vi "Drive Controller.vi"(8 "error in":errorcluster) -> ()   [LabVIEW 2015]
doc: "This VI executes continuously carrying out the current operation and responding to updates or new operation requests. It will often contain the timing or control code that is difficult to place directly in TeleOp. This VI generally opens all sensors and motors and isolates the rest of the robot code from knowing implementation details of how the operations are carried out."
uses:
  Drive Operations.ctl
  Drive Setpoints.ctl
  <vilib>/Rock Robotics/WPI/SafetyOutput/WPI_SafetyOutputConfigMenu.ctl
  Support Code/Team900-VIs/navX/navX Library v2/navX Library v2.lvlib
  Support Code/Team900-VIs/Team900SwerveDrive/Team900SwerveDrive.lvlib
  <vilib>/Rock Robotics/WPI/RobotDrive/WPI_RobotDriveOpen4MotorWithCANTalonSRX.vi
  Support Code/Team900-VIs/navX/navX Library v2/IO/Open/Z900_navX_Open_SPI.vi
  <vilib>/Rock Robotics/SystemInterfaces/spilib/spi_bus.ctl
panel:
  out "Setpoints":T1(graph)
  out "Current\nCmd":string
  # "Tip: It may be helpful to observe inputs and sensor values.\nYou may also want to display tuning or debugging controls."
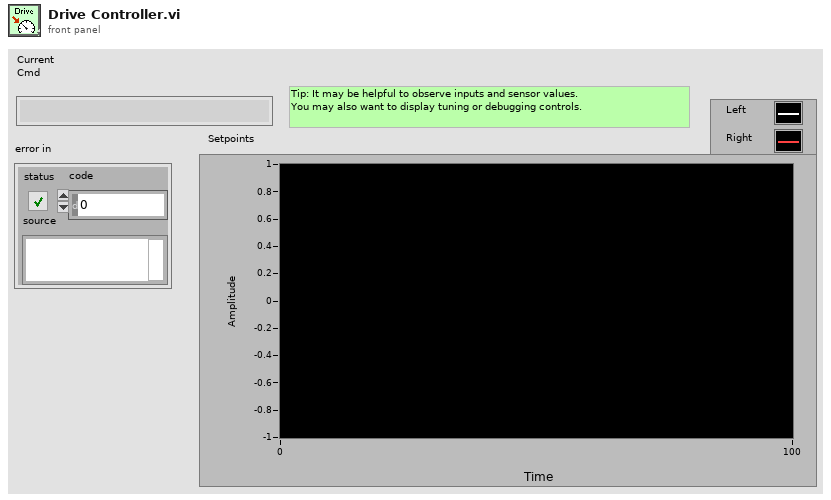
[diagram p1: front panel]
types:
  T1 = cluster{"Left Setpoint":dbl, "Right Setpoint":dbl}
  T2 = typedef "spi_bus.ctl" = enum16{"SPI On-Board, CS0", "SPI On-Board, CS1", "SPI On-Board, CS2", "SPI On-Board, CS3", "SPI MXP", "Invalid"}
  T3 = typedef "WPI_SafetyOutputConfigMenu.ctl" = enum16{"Enable", "Disable"}
  T4 = typedef "Drive Setpoints.ctl" = cluster{"Operation":T5, "Left Setpoint":dbl, "Right Setpoint":dbl, "Duration":dbl, "Straight Setpoint":dbl}
  T5 = typedef "Drive Operations.ctl" = enum16{"Reserve", "Read Current", "Immediate", "Drive for Time", "Drive for Distance", "Cross Defense"}
  T6 = typedef "WPI_RobotDriveDevRef.ctl" = cluster{"DevStatus":errorcluster, "Motors[]":T7[], "Square Inputs":bool, "Max Output":dbl}
  T7 = typedef "WPI_MotorControlDeviceRef.ctl" = cluster{"DeviceStatus":errorcluster, "Type":T8, "PWM":cluster{"PWM Channel":T9, "DeadBand":T10}, "CAN":cluster{"Device Number":u8, "Control Mode":T11, "Semaphore":T12, "Max Vout":dbl, "TalonSRX Control Mode":T13}, "Invert":bool}
  T8 = typedef "WPI_MotorControlType.ctl" = enum16{"PWM", "CAN", "CANTalonSRX"}
  T9 = typedef "FPGA_DIOPWMChannel.ctl" = enum8{"PWM 0", "PWM 1", "PWM 2", "PWM 3", "PWM 4", "PWM 5", "PWM 6", "PWM 7", "PWM 8", "PWM 9", "PWM MXP 0", "PWM MXP 1", "PWM MXP 2", "PWM MXP 3", "PWM MXP 4", "PWM MXP 5", "PWM MXP 6", "PWM MXP 7", "PWM MXP 8", "PWM MXP 9", "Invalid"}
  T10 = typedef "WPI_PWMDeadband.ctl" = cluster{"Name":string, "maxPositivePwm":i32, "minPositivePwm":i32, "centerPwm":i32, "maxNegativePwm":i32, "minNegativePwm":i32, "angularRange":u16}
  T11 = typedef "WPI_CANJaguar_ControlMode.ctl" = enum8{"Percent VBus", "Current", "Speed", "Position", "Voltage"}
  T12 = typedef "Semaphore RefNum" = refnum<k1>
  T13 = typedef "WPI_CANTalonSRX_APIControlMode.ctl" = enum8{"Percent VBus", "Speed", "Position", "Slave", "Unchanged / Invalid", "Voltage Compensation", "Current", "Motion Profile"}
  T14 = typedef "navX Library v2.lvlib/Z900_navX_DeviceTypeDef.ctl" = cluster{"Interface":cluster{"Protocol":T15, "Update Rate (4Hz-60Hz)":u8, "navX Open TypeDef":variant}, "Notify Packet":refnum<notifier>, "Loop VI Refnum":refnum<vi>, "Ready to Close Occurrence Refnum":refnum<k4>}
  T15 = typedef "navX Library v2.lvlib/Z900_navX_ProtocolTypeDef.ctl" = enum16{"SERIAL", "I2C", "SPI"}
  T16 = cluster{"Velocity X":dbl, "Velocity Y":dbl, "Velocity Z":dbl, "Displacement X":dbl, "Displacement Y":dbl, "Displacement Z":dbl}
  T17 = typedef "Command Status Info.ctl" = cluster{"Name":string, "Status":T18, "notifier out":T19}
  T18 = typedef "Completion Status.ctl" = enum16{"Successful", "Aborted", "Incomplete"}
  T19 = typedef "Completion Notifier.ctl" = refnum<notifier>
  T20 = cluster{"SubSystem Data":T4, cluster{"Start Time (ms)":u32, "Iterations":i32}, cluster{"Command Info":T17, "Description":string, "SubSystem Data":T4, "notifier out":refnum<notifier>, "Subsystem Name":string}}
  T21 = cluster{"Yaw":dbl, "Roll":dbl, "Pitch":dbl, "Heading":dbl, "Fused Heading":dbl}
  T22 = cluster{"Don't move motors while reserved":dbl, "Don't move motors while reserved":dbl}
  T23 = cluster{"SubSystem Data":T4, cluster{"Start Time (ms)":u32, "Iterations":i32}, "Default Command Arguments":cluster{"Command Info":T17, "Description":string, "SubSystem Data":T4, "notifier out":refnum<notifier>, "Subsystem Name":string}}
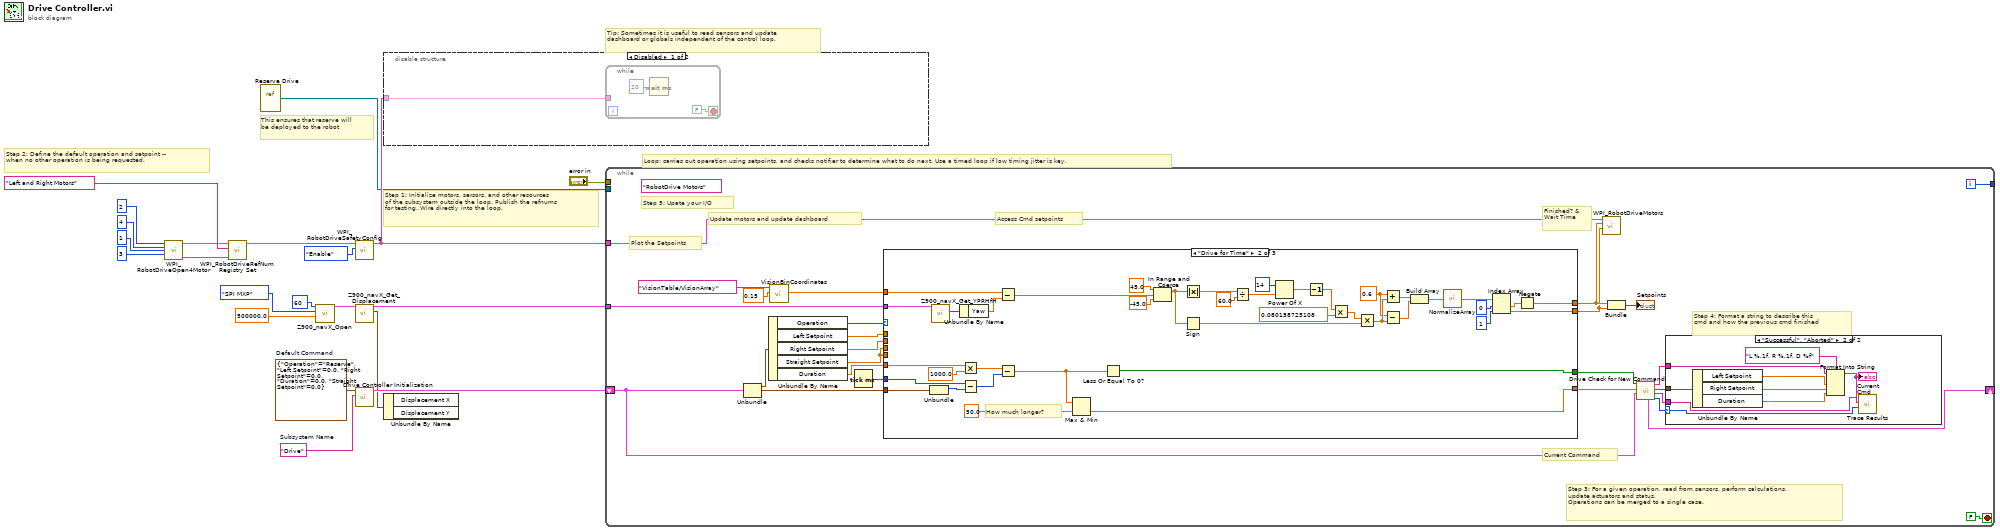
[diagram p0: block diagram]
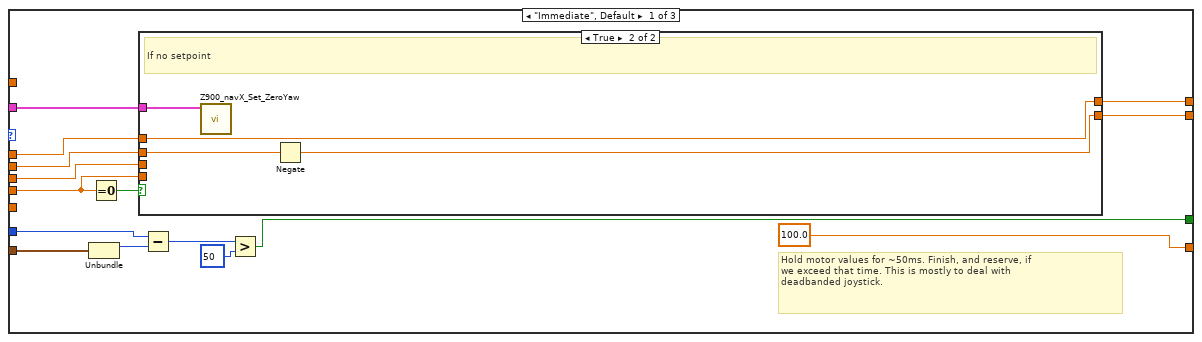
[diagram p4: hidden frame]
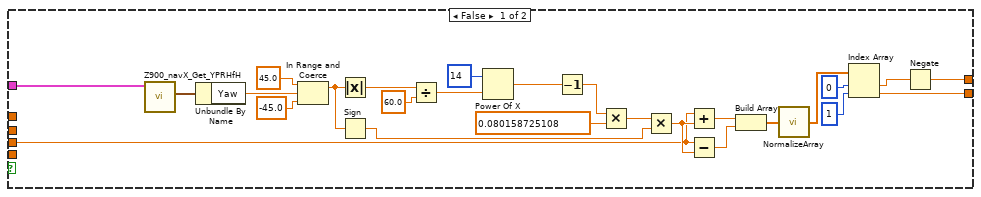
[diagram p5: hidden frame]
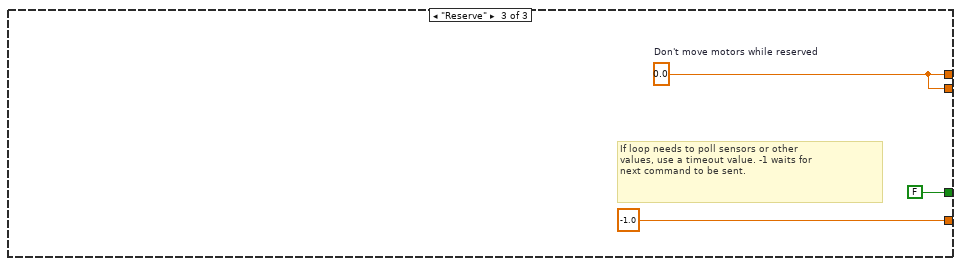
[diagram p6: hidden frame]
diagram:
  w20 = T4 {"Operation"=enum."Reserve", "Left Setpoint"=0.0, "Right Setpoint"=0.0, "Duration"=0.0, "Straight Setpoint"=0.0}  # Default Command
  w21 = "Drive"  # Subsystem Name
  # "This ensures that reserve will\nbe deployed to the robot"
  # "Tip: Sometimes it is useful to read sensors and update\ndashboard or globals independent of the control loop."
  # "Step 2: Define the default operation and setpoint --\nwhen no other operation is being requested."
  # "Step 1: Initialize motors, sersors, and other resources\nof the subsystem outside the loop. Publish the refnums\nfor testing. Wire directly into the loop."
  # "Loop: carries out operation using setpoints, and checks notifier to determine what to do next. Use a timed loop if low timing jitter is key."
  n1 = call-poly <vilib>:"WPI_RobotDriveOpen4Motor.vi"("Rear Left Motor"=u8 2, "Rear Right Motor"=u8 4, "Front Left Motor"=u8 1, "Front Right Motor"=u8 3) -> ("RobotDriveDevRef"=w12:T6, "error out"=w11:errorcluster)  [unwired: 10 in]
  n2 = call <vilib>:"WPI_RobotDriveRefNum Registry Set.vi"("error in (no error)"=w11, "refnum name"="Left and Right Motors", "RobotDriveDevRef"=w12) -> ("RobotDriveDevRef"=w18:T6)  [unwired: 1 in, 7 out]
  n3 = vi-ref "Reserve Drive.vi"() -> (w13:refnum<vi>)
  n4 = call-poly "Z900_navX_Open.vi"("Clock Rate (Hz)"=500000.0, "SPI Bus"=spi_bus."SPI MXP", "Update Rate (4Hz-60Hz)"=u8 60) -> ("navX Device"=w3:T14)  [unwired: 7 in, 1 out]
  n5 = call <vilib>:"WPI_RobotDriveSafetyConfig.vi"("mode"=WPI_SafetyOutputConfigMenu."Enable", "RobotDriveDevRef"=w18) -> ("RobotDriveDevRef"=w16:T6)  [unwired: 8 in, 1 out]
  n6 = call "Z900_navX_Get_Displacement.vi"("navX Device"=w3) -> ("Displacement"=w1:T16, "navX Device"=w2:T14)  [unwired: 7 in, 2 out]
  n7 = call "Drive Controller Initialization.vi"("Subsystem Name"=w21, "Default Command"=w20) -> ("output cluster"=w14:T20)  [unwired: 9 in]
  n8 = disable-structure shown="Disabled" {
    disable-tunnel: w16 -> [w22 _]
    frame Disabled {
      n9 = while {
        tunnel: w22 -> [_]
        stop <- FALSE stop-if-true
        n10 = Wait (ms)(milliseconds to wait=u32 20) -> ()  [unwired: 1 out]
      }
    }
    frame Enabled {
    }
  }
  n11 = Unbundle By Name(w1) -> ()  [unwired: 2 out]
  n12 = while {
    shift-right: [w38] -> _
    shift-left: w14 -> [w31]
    tunnel: [w49] -> _
    tunnel: w16 -> [w45]
    tunnel: "error in" -> [_]
    tunnel: w13 -> [_]
    tunnel: w2 -> [w28]
    i -> [w49]
    stop <- FALSE stop-if-true
    (unwired) "RobotDrive Motors" ("Name")
    # "Step 5: Upate your I/O"
    # "Step 4: Format a string to describe this\ncmd and how the previous cmd finished"
    # "Current Command"
    # "Update motors and update dashboard"
    # "Plot the Setpoints"
    # "Access Cmd setpoints"
    # "Finished? &\nWait Time"
    # "Step 3: For a given operation, read from sensors, perform calculations,\nupdate actuators and status.\nOperations can be merged to a single case."
    n13 = Unbundle(w31) -> ("SubSystem Data"=w44:T4, w32:cluster{"Start Time (ms)":u32, "Iterations":i32})  [unwired: 1 out]
    n14 = Unbundle By Name(w44) -> ("Operation"=w43:T5, "Left Setpoint"=w42:dbl, "Right Setpoint"=w41:dbl, "Straight Setpoint"=w29:dbl, "Duration"=w30:dbl)
    n15 = call "VisionBinCoordinates.vi"("Minimum Ratio"=0.15, "Vision Array Name"="VisionTable/VisionArray") -> ("bin angle"=w25:dbl)  [unwired: 2 in, 4 out]
    n16 = Tick Count (ms)() -> (millisecond timer value=w40:u32)
    n17 = case shown="\"Drive for Time\"" w43 {
      tunnel: [100.0 w134 -1.0] -> w37
      tunnel: [w69 w138 FALSE ("ignore previous (F)")] -> w36
      tunnel: w32 -> [w68 w140 _]
      tunnel: [w66 w110 w144] -> w47
      tunnel: [w64 w111 w144] -> w46
      tunnel: w42 -> [w65 _ _]
      tunnel: w41 -> [w63 _ _]
      tunnel: w29 -> [w62 _ _]
      tunnel: w40 -> [w70 w137 _]
      tunnel: w30 -> [_ w133 _]
      tunnel: w28 -> [w61 w108 _]
      tunnel: w29 -> [w60 _ _]
      tunnel: w25 -> [_ w105 _]
      frame "Immediate", Default {
        # "Hold motor values for ~50ms. Finish, and reserve, if\nwe exceed that time. This is mostly to deal with\ndeadbanded joystick."
        n18 = Unbundle(w68) -> ("Start Time (ms)"=w71:u32)  [unwired: 1 out]
        n19 = Equal To 0?(x=w62) -> (x = 0?=w67:bool)
        n20 = case shown="True" w67 {
          tunnel: [w80 w104] -> w66
          tunnel: w65 -> [_ w104]
          tunnel: [w81 w101] -> w64
          tunnel: w63 -> [_ w103]
          tunnel: w62 -> [_ _]
          tunnel: w61 -> [w100 w102]
          tunnel: w60 -> [w84 _]
          frame False {
            n21 = call "Z900_navX_Get_YPRHfH.vi"("navX Device"=w100) -> ("YRPHfH"=w83:T21)  [unwired: 7 in, 3 out]
            n22 = Unbundle By Name(w83) -> ("Yaw"=w76:dbl)
            n23 = In Range and Coerce(upper limit=45.0, x=w76, lower limit=-45.0) -> (coerced(x)=w75:dbl)  [unwired: 1 out]
            n24 = Absolute Value(x=w75) -> (abs(x)=w94:dbl)
            n25 = Sign(1:w75) -> (0:w92:dbl)
            n26 = Divide(x=w94, y=60.0) -> (x/y=w97:dbl)
            n27 = Power Of X(1:w97, 2:14) -> (0:w96:dbl)
            n28 = Decrement(x=w96) -> (x-1=w95:dbl)
            n29 = Multiply(x=w95, y=0.080158725108) -> (x*y=w93:dbl)
            n30 = Multiply(x=w93, y=w92) -> (x*y=w91:dbl)
            n31 = Add(x=w84, y=w91) -> (x+y=w86:dbl)
            n32 = Subtract(x=w84, y=w91) -> (x-y=w85:dbl)
            n33 = Build Array(w86, w85) -> (w90:dbl[])
            n34 = call "NormalizeArray.vi"("array"=w90) -> ("normalized array"=w89:dbl[])
            n35 = Index Array(array=w89, index #1=0 ("index"), index #2=1 ("index")) -> (element #1=w82:dbl, element #2=w81:dbl)
            n36 = Negate(x=w82) -> (-x=w80:dbl)
          }
          frame True {
            # "If no setpoint"
            n37 = call "Z900_navX_Set_ZeroYaw.vi"("navX Device"=w102) -> ()  [unwired: 9 in, 2 out]
            n38 = Negate(x=w103) -> (-x=w101:dbl)
          }
        }
        n39 = Subtract(x=w70, y=w71) -> (x-y=w72:u32)
        n40 = Greater?(x=w72, y=u8 50 ("Left Motor")) -> (0:w69:bool)
      }
      frame "Drive for Time" {
        w109 = 0.6
        # "How much longer?"
        n41 = Unbundle(w140) -> ("Start Time (ms)"=w139:u32)  [unwired: 1 out]
        n42 = call "Z900_navX_Get_YPRHfH.vi"("navX Device"=w108) -> ("YRPHfH"=w117:T21)  [unwired: 7 in, 3 out]
        n43 = Unbundle By Name(w117) -> ("Yaw"=w107:dbl)
        n44 = Multiply(x=w133, y=1000.0) -> (x*y=w142:dbl)
        n45 = Subtract(x=w137, y=w139) -> (x-y=w143:u32)
        n46 = Subtract(x=w105, y=w107) -> (x-y=w106:dbl)
        n47 = Subtract(x=w142, y=w143) -> (x-y=w136:dbl)
        n48 = Max & Min(x=w136, y=50.0) -> (min(x,y)=w134:dbl)  [unwired: 1 out]
        n49 = Less Or Equal To 0?(x=w136) -> (x <= 0?=w138:bool)
        n50 = In Range and Coerce(upper limit=45.0, x=w106, lower limit=-45.0) -> (coerced(x)=w112:dbl)  [unwired: 1 out]
        n51 = Absolute Value(x=w112) -> (abs(x)=w127:dbl)
        n52 = Sign(1:w112) -> (0:w125:dbl)
        n53 = Divide(x=w127, y=60.0) -> (x/y=w130:dbl)
        n54 = Power Of X(1:w130, 2:14) -> (0:w129:dbl)
        n55 = Decrement(x=w129) -> (x-1=w128:dbl)
        n56 = Multiply(x=w128, y=0.080158725108) -> (x*y=w126:dbl)
        n57 = Multiply(x=w126, y=w125) -> (x*y=w124:dbl)
        n58 = Add(x=w109, y=w124) -> (x+y=w119:dbl)
        n59 = Subtract(x=w109, y=w124) -> (x-y=w118:dbl)
        n60 = Build Array(w119, w118) -> (w123:dbl[])
        n61 = call "NormalizeArray.vi"("array"=w123) -> ("normalized array"=w122:dbl[])
        n62 = Index Array(array=w122, index #1=0 ("index"), index #2=1 ("index")) -> (element #1=w116:dbl, element #2=w111:dbl)
        n63 = Negate(x=w116) -> (-x=w110:dbl)
      }
      frame "Reserve" {
        w144 = 0.0  # Don't move motors while reserved
        # "If loop needs to poll sensors or other\nvalues, use a timeout value. -1 waits for\nnext command to be sent."
      }
    }
    n64 = call <vilib>:"WPI_RobotDriveMotors.vi"("RightSpeed"=w46, "LeftSpeed"=w47, "RobotDriveDevRef"=w45) -> ()  [unwired: 1 in, 8 out]
    n65 = Bundle("Don't move motors while reserved"=w47, "Don't move motors while reserved"=w46) -> (→"Setpoints":T22)  [unwired: 1 in]
    n66 = call "Drive Check for New Command.vi"("input cluster"=w31, "Wait time (ms)"=w37, "Finished?"=w36) -> ("Completion"=w39:T18, "Subsystem Name"=w33:string, "SetPoint"=w34:T4, "Initial Trace String"=w35:string, "output cluster"=w38:T23)  [unwired: 4 in]
    n67 = case shown="\"Successful\", \"Aborted\"" w39 {
      selector: w39 -> [_ w59]
      tunnel: w35 -> [_ w54]
      tunnel: w34 -> [_ w55]
      tunnel: w33 -> [_ w51]
      frame "Incomplete", Default {
        # "Continuing current command"
      }
      frame "Successful", "Aborted" {
        # "Report and setup for next command"
        n68 = Unbundle By Name(w55) -> ("Left Setpoint"=w57:dbl, "Right Setpoint"=w58:dbl, "Duration"=w52:dbl)
        n69 = Format Into String(format string="L %.1f, R %.1f, D %f", initial string=w54, w57, w58, w52) -> (resulting string=w53:string)  [unwired: 1 in, 1 out]
        "Current\nCmd" <- w53
        n70 = call <vilib>:"Trace Results.vi"("Status of previous command"=w59, "Description"=w53, "Subsystem"=w51) -> ()  [unwired: 9 in]
      }
    }
  }
